vi "Get Software Feeds.vi"(8 "error in (no error)":errorcluster, 11 "Session in":refnum<k21>) -> (0 "error out":errorcluster, 2 "Software Feeds":T1[](array[typedef]), 3 "Session out":refnum<k21>)   [LabVIEW 2020, in "nisyscfg.lvlib"]
doc: "Retrieves a list of software feeds installed on a system. A software feed has a name and location (URI) that identifies a source from which packages can be installed."
uses:
  <vilib>/nisyscfg/nisyscfg.lvlib
  <vilib>/nisyscfg/Software Feed.ctl
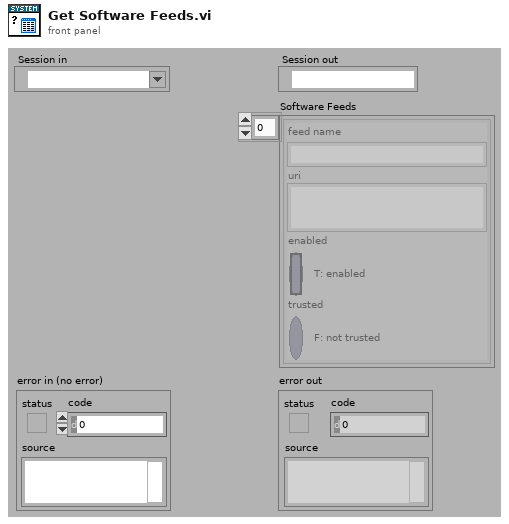
[diagram p1: front panel]
types:
  T1 = typedef "nisyscfg.lvlib/Software Feed.ctl" = cluster{"feed name":string, "uri":string, "enabled":bool, "trusted":bool}
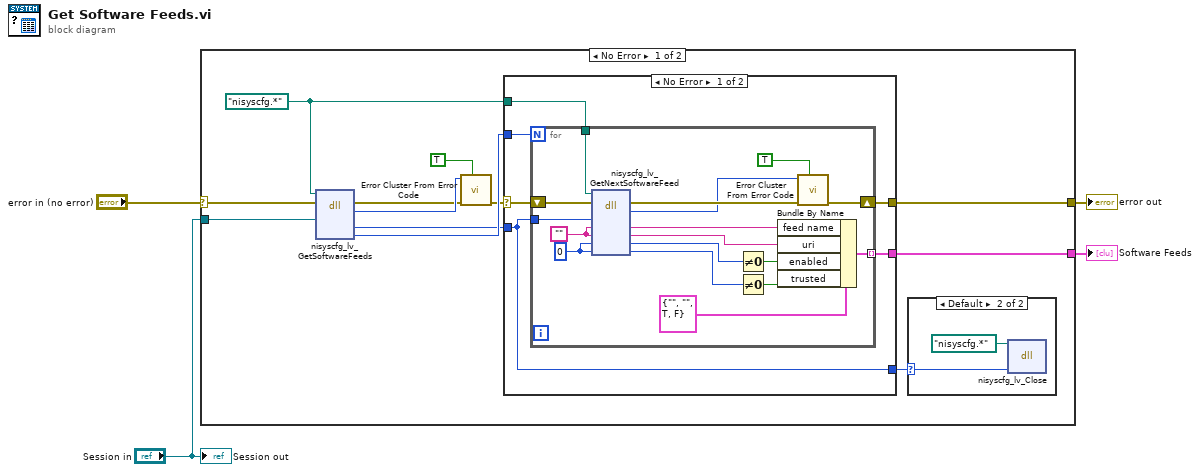
[diagram p0: block diagram]
diagram:
  n1 = case shown="No Error" "error in (no error)" {
    selector: "error in (no error)" -> [w15 w43]
    tunnel: [w8 w43] -> w4
    tunnel: "Session in" -> [w14 _]
    tunnel: [w7 _] -> w1
    frame No Error {
      w6 = path "nisyscfg.*" ("path in")
      n2 = dll-call lib="nisyscfg.*" fn="nisyscfg_lv_GetSoftwareFeeds" label="GetSoftwareFeeds"(path in=w6, error in=w15, "system"=w14) -> (error out=w12:errorcluster, "result"=w16:i32, "feeds"=w10:u64, "numFeeds"=w11:i32)  [unwired: 4 in, 1 out]
      n3 = call <vilib>:"Error Cluster From Error Code.vi"("show call chain? (False)"=TRUE, "error in (no error)"=w12, "error code (0)"=w16) -> ("error out"=w9:errorcluster)  [unwired: 6 in]
      n4 = case shown="No Error" w9 {
        selector: w9 -> [w24 w42]
        tunnel: [w23 w42] -> w8
        tunnel: w10 -> [w19 _]
        tunnel: w11 -> [w22 _]
        tunnel: [w21 _] -> w7
        tunnel: w6 -> [w20 _]
        tunnel: [w19 _] -> w5
        frame No Error {
          n5 = for {
            N: w22 -> [_]
            shift-right: [w28] -> w23
            shift-left: w24 -> [w40]
            tunnel: w19 -> [w41]
            tunnel: [w32] -> w21 mode=indexing
            tunnel: w20 -> [w25]
            w26 = ""
            w27 = u8 0 ("enabled")
            n6 = dll-call lib="nisyscfg.*" fn="nisyscfg_lv_GetNextSoftwareFeed" label="GetNextSoftwareFeed"(path in=w25, error in=w40, "feedEnum"=w41, "feedName"=w26, "uri"=w26, "enabled"=w27, "trusted"=w27) -> (error out=w30:errorcluster, "result"=w29:i32, "feedName"=w38:string, "uri"=w37:string, "enabled"=w34:u8, "trusted"=w33:u8)  [unwired: 2 in, 1 out]
            n7 = Not Equal To 0?(x=w34) -> (x != 0?=w36:bool)
            n8 = Not Equal To 0?(x=w33) -> (x != 0?=w35:bool)
            n9 = Bundle By Name(cluster=T1 {"feed name"="", "uri"="", "enabled"=TRUE, "trusted"=FALSE} ("software feed"), "feed name"=w38, "uri"=w37, "enabled"=w36, "trusted"=w35) -> (w32:T1)
            n10 = call <vilib>:"Error Cluster From Error Code.vi"("show call chain? (False)"=TRUE, "error in (no error)"=w30, "error code (0)"=w29) -> ("error out"=w28:errorcluster)  [unwired: 6 in]
          }
        }
        frame Error {
        }
      }
      n11 = case shown="Default" w5 {
        selector: w5 -> [_ w17]
        frame 0 {
          # "No need to call Close\non an empty enum."
        }
        frame Default {
          n12 = dll-call lib="nisyscfg.*" fn="nisyscfg_lv_Close" label="Close"(path in=path "nisyscfg.*", "expertsEnum"=w17) -> ()  [unwired: 3 in, 3 out]
        }
      }
    }
    frame Error {
    }
  }
  "error out" <- w4
  "Software Feeds" <- w1
  "Session out" <- "Session in"
